vi "Properties-Set Public.vi"(1 "Variant":variant, 2 "New Public":T1) -> (0 "Variant 2":variant)   [LabVIEW 2019]
uses:
  Sub Controls/Public.ctl
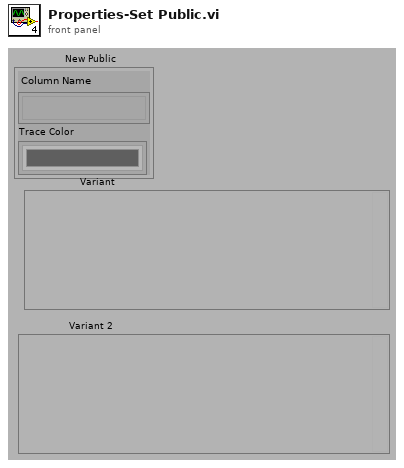
[diagram p1: front panel]
types:
  T1 = typedef "Public.ctl" = cluster{"Column Name":string[], "Trace Color":u32[]}
  T2 = typedef "Instrument Properties.ctl" = cluster{"Public":T1, "Private":T3}
  T3 = typedef "Private.ctl" = cluster{"Path":path, "VI Refnum":T4, "Name":string, "# of Values":i32, "Scale Factors":dbl[], "Display":T5[], "Offset":dbl[]}
  T4 = typedef "Instrument Ref.ctl" = refnum<vi>
  T5 = typedef "SystemCheckBox-resize.ctl" = bool
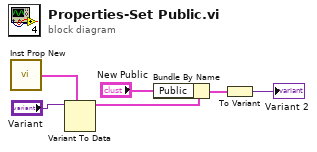
[diagram p0: block diagram]
diagram:
  n1 = call "Inst Prop New.vi"() -> ("Instrument Prop Out"=w5:T2)
  n2 = Variant To Data(type=w5, Variant="Variant") -> (data=w3:T2)  [unwired: 1 in, 1 out]
  n3 = Bundle By Name(cluster=w3, "Public"="New Public") -> (w2:T2)
  n4 = To Variant(anything=w2) -> (Variant=→"Variant 2":variant)
